vi "CityInBottle_Interpolated (1).vi"() -> ()   [LabVIEW 2024]
uses:
  <vilib>/gmath/interp.llb/Interpolate 2D (2d X,Y).vi
  <vilib>/gmath/NI_Gmath.lvlib
panel:
  in  "ms wait":u32(slide)=50 scale=1.0..100.0
  in  "Texture OFF":bool
  in  "Texture":bool
  in  "Building Depth":i32(slide)=8 caption="Building Depth\n(8)" scale=0.0..100.0
  out "Time/Frame":i32=48
  in  "Ground Plane":i32(slide)=6 caption="Ground Plane\n(6)" scale=90.0..1.0
  in  "Avenue Period":i32(slide)=99 caption="Avenue Period\n(99)" scale=25.0..175.0
  in  "Building Height":i32(slide)=45 caption="Building Height\n(46)" scale=0.0..100.0
  in  "Building Width":i32(slide)=9 caption="Building Width\n(9)" scale=0.0..100.0
  in  "Avenue Width":i32(slide)=27 caption="Avenue Width\n(27)" scale=1.0..100.0
  in  "City Distance":i32(slide)=32 caption="City Distance\n(32)" scale=1.0..100.0
  in  "background":bool
  in  "Stop":bool
  out "City\nin\nBottle":dbl[][](graph) caption="City in Graph"
  # "A City in a Bottle"
  # "Inspired by Frank Force"
  # "https://capjs.3d2k.com"
  # "Original Source Code"
  # "t*=60\nfor(c.width=w=99,++t,i=6e3;i--;c.getContext`2d`.fillRect(i%w,i/w|0,1-d*Z/w+s,1))for(a=i%w/50-1,s=b=1-i/4e3,X=t,Y=Z=d=1;++Z<w&(Y<6-(32<Z&27<X%w&&X/9^Z/8)*8%46||d|(s=(X&Y&Z)%3/Z,a=b=1,d=Z/w));Y-=b)X+=a"
  # "https://observablehq.com/@darabos/decoding-a-city-in-a-bottle"
  # "https://frankforce.com/city-in-a-bottle-a-256-byte-raycasting-system/"
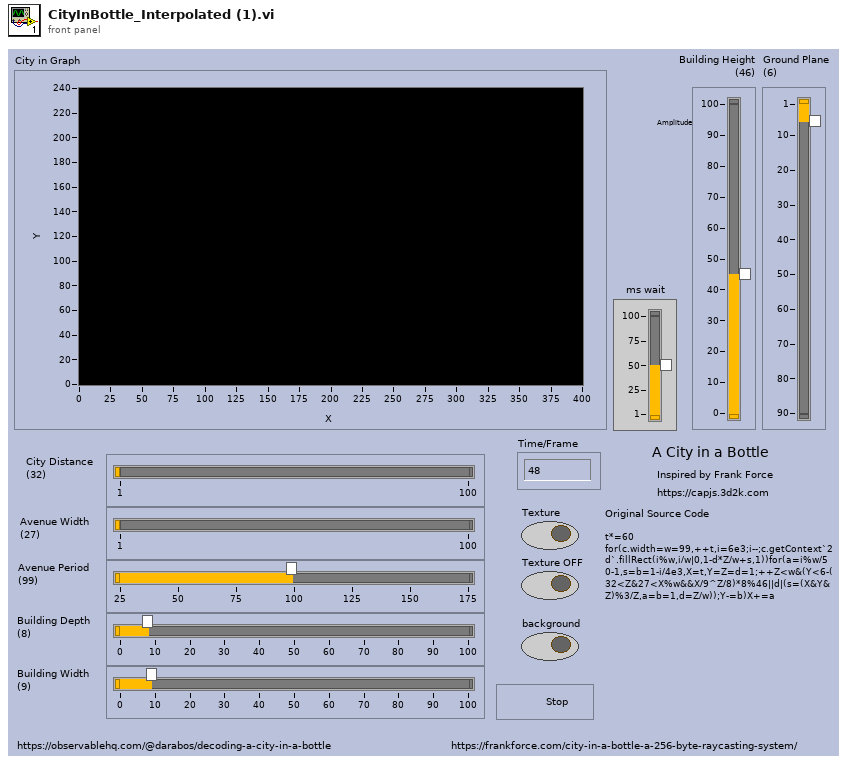
[diagram p1: front panel]
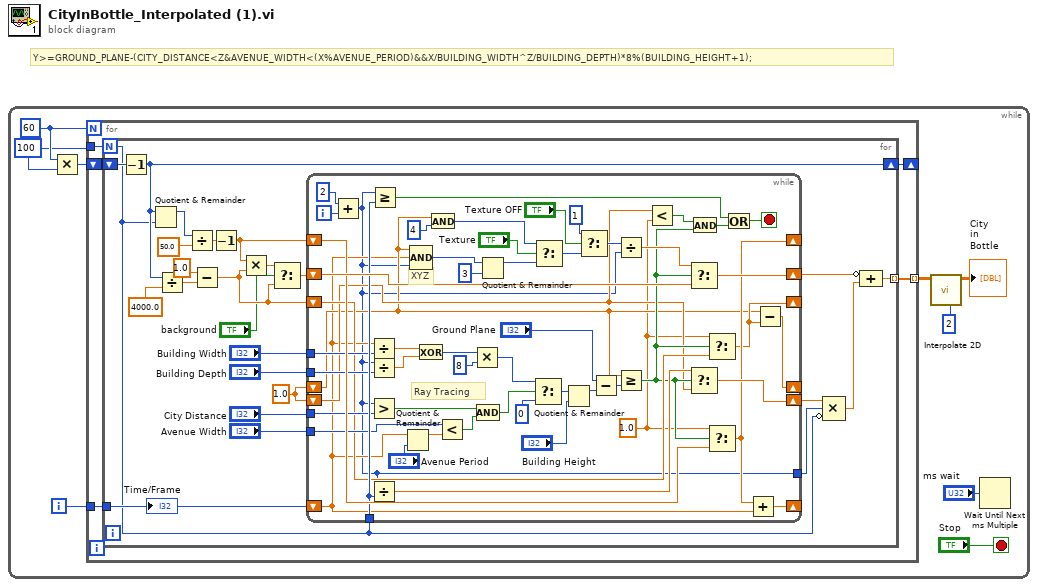
[diagram p0: block diagram]
diagram:
  # "Y>=GROUND_PLANE-(CITY_DISTANCE<Z&AVENUE_WIDTH<(X%AVENUE_PERIOD)&&X/BUILDING_WIDTH^Z/BUILDING_DEPTH)*8%(BUILDING_HEIGHT+1);"
  n1 = while {
    i -> [w8]
    stop <- "Stop" stop-if-true
    w4 = 100
    w6 = 60
    n2 = Multiply(x=w6, y=w4) -> (x*y=w5:i32)
    n3 = for {
      N: w6 -> [_]
      tunnel: [w11] -> w3 mode=indexing
      tunnel: w8 -> [w14]
      shift-right: [w12] -> _
      shift-left: w5 -> [w13]
      tunnel: w4 -> [w10]
      n4 = for {
        N: w10 -> [w16]
        tunnel: [w17] -> w11 mode=indexing
        tunnel: w14 -> [w21]
        shift-right: [w19] -> w12
        shift-left: w13 -> [w20]
        w23 = sgl 1.0 ("d")
        n5 = Decrement(x=w20) -> (x-1=w19:i32)
        n6 = Quotient & Remainder(x=w19, y=w16) -> (x-y*floor(x/y)=w28:i32)  [unwired: 1 out]
        n7 = Divide(x=w19, y=sgl 4000.0) -> (x/y=w36:sgl)
        n8 = Divide(x=w28, y=sgl 50.0) -> (x/y=w38:sgl)
        n9 = Subtract(x=sgl 1.0, y=w36) -> (x-y=w32:sgl)
        n10 = Decrement(x=w38) -> (x-1=w33:sgl)
        n11 = Multiply(x=w33, y=w32) -> (x*y=w34:sgl)
        n12 = Select(t=w34, s="background", f=w32) -> (s? t:f=w31:sgl)
        n13 = while {
          tunnel: w16 -> [w85]
          shift-right: [w90] -> _
          shift-left: w23 -> [w48]
          shift-right: [w91] -> _
          shift-left: w21 -> [w47]
          shift-right: [w77] -> w30
          shift-left: w23 -> [w62]
          shift-right: [w70] -> _
          shift-left: w33 -> [w86]
          shift-right: [w69] -> _
          shift-left: w32 -> [w76]
          shift-right: [w89] -> w18
          shift-left: w31 -> [w87]
          tunnel: "City Distance" -> [w82]
          tunnel: "Avenue Width" -> [w81]
          tunnel: "Building Width" -> [w80]
          tunnel: "Building Depth" -> [w79]
          tunnel: [w40] -> w29
          i -> [w93]
          stop <- w73 stop-if-true
          w45 = sgl 1.0 ("y")
          # "Ray Tracing"
          # "XYZ"
          n14 = Add(x=2, y=w93) -> (x+y=w40:i32)
          n15 = Divide(x=w47, y=w80) -> (x/y=w43:sgl)
          n16 = Divide(x=w40, y=w79) -> (x/y=w42:dbl)
          n17 = Greater?(x=w40, y=w82) -> (0:w58:bool)
          n18 = Divide(x=w40, y=w85) -> (x/y=w78:sgl)
          n19 = Greater Or Equal?(x=w40, y=w85) -> (x >= y?=w72:bool)
          n20 = Quotient & Remainder(x=w47, y="Avenue Period") -> (x-y*floor(x/y)=w46:sgl)  [unwired: 1 out]
          n21 = Compound Arithmetic op=AND(w48, w47, w40) -> (w84:i32)
          n22 = Exclusive Or(1:w42, 2:w43) -> (0:w56:i32)
          n23 = And(x=w48, y=4) -> (x .and. y?=w67:i32)
          n24 = Less?(x=w81, y=w46) -> (x < y?=w57:bool)
          n25 = Multiply(x=w56, y=8) -> (x*y=w55:i32)
          n26 = Compound Arithmetic op=AND(w58, w57) -> (w44:bool)
          n27 = Quotient & Remainder(x=w84, y=3) -> (x-y*floor(x/y)=w66:i32)  [unwired: 1 out]
          n28 = Select(t=w55, s=w44, f=0) -> (s? t:f=w54:i32)
          n29 = Select(t=w67, s="Texture", f=w66) -> (s? t:f=w65:i32)
          n30 = Quotient & Remainder(x=w54, y="Building Height") -> (x-y*floor(x/y)=w59:i32)  [unwired: 1 out]
          n31 = Select(t=1, s="Texture OFF", f=w65) -> (s? t:f=w63:i32)
          n32 = Subtract(x="Ground Plane", y=w59) -> (x-y=w41:i32)
          n33 = Divide(x=w63, y=w40) -> (x/y=w88:sgl)
          n34 = Greater Or Equal?(x=w48, y=w41) -> (x >= y?=w74:bool)
          n35 = Less?(x=w62, y=w45) -> (x < y?=w71:bool)
          n36 = Select(t=w88, s=w74, f=w87) -> (s? t:f=w89:sgl)
          n37 = Select(t=w78, s=w74, f=w62) -> (s? t:f=w77:sgl)
          n38 = And(x=w71, y=w74) -> (x .and. y?=w75:bool)
          n39 = Select(t=w45, s=w74, f=w76) -> (s? t:f=w69:sgl)
          n40 = Select(t=w45, s=w74, f=w86) -> (s? t:f=w70:sgl)
          n41 = Or(x=w72, y=w75) -> (x .or. y?=w73:bool)
          n42 = Add(x=w70, y=w47) -> (x+y=w91:sgl)
          n43 = Subtract(x=w48, y=w69) -> (x-y=w90:sgl)
        }
        n44 = Compound Arithmetic op=MULTIPLY(w30, w29, invert w16) -> (w15:dbl)
        n45 = Compound Arithmetic op=ADD(invert w18, w15) -> (w17:dbl)
        "Time/Frame" <- w21
      }
    }
    n46 = call-poly <vilib>:"Interpolate 2D.vi"("ntimes"=2, "Z"=w3) -> ("zi"=→"City\nin\nBottle":dbl[][])  [unwired: 6 in, 3 out]
    n47 = Wait Until Next ms Multiple(millisecond multiple="ms wait") -> ()  [unwired: 1 out]
  }
